vi "Fundamental Phasors.vi"(8 "error in (no error)":errorcluster, 10 "current waveform":waveform(dbl), 11 "voltage waveform":waveform(dbl)) -> (0 "error out":errorcluster, 1 "frequency":dbl, 2 "current fundamental vector":cdb, 3 "voltage fundamental vector":cdb)   [LabVIEW 2021]
uses:
  <vilib>/measure/matone.llb/Extract Single Tone Information 1 Chan.vi
  <vilib>/measure/NI_MAPro.lvlib
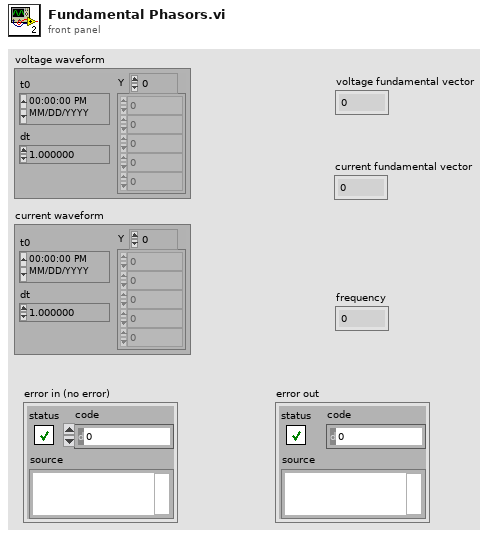
[diagram p1: front panel]
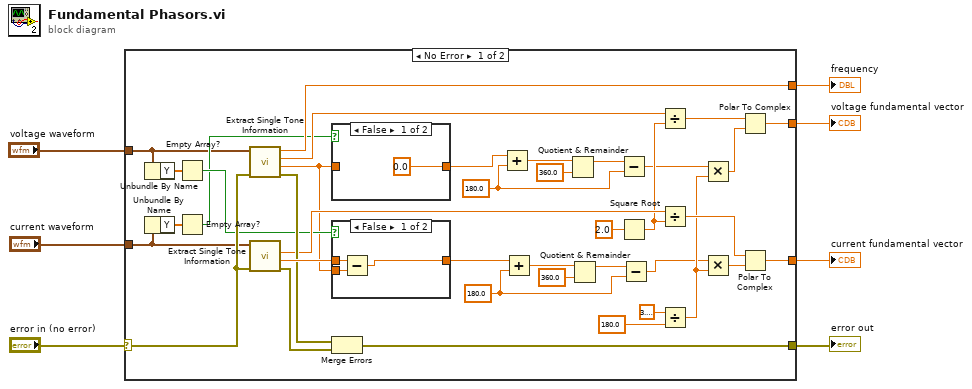
[diagram p0: block diagram]
diagram:
  n1 = case shown="No Error" "error in (no error)" {
    selector: "error in (no error)" -> [w40 w52]
    tunnel: "voltage waveform" -> [w20 _]
    tunnel: [w31 w52] -> w2
    tunnel: [w42 _] -> w6
    tunnel: [w41 _] -> w3
    tunnel: "current waveform" -> [w21 _]
    tunnel: [w34 _] -> w4
    frame No Error {
      w10 = 180.0 ("x")
      w16 = 180.0 ("x")
      n2 = Unbundle By Name(w20) -> ("Y"=w29:dbl[])
      n3 = Unbundle By Name(w21) -> ("Y"=w27:dbl[])
      n4 = Empty Array?(array=w29) -> (empty?=w28:bool)
      n5 = Empty Array?(array=w27) -> (empty?=w26:bool)
      n6 = call-poly <vilib>:"Extract Single Tone Information.vi"("error in (no error)"=w40, "time signal in"=w20) -> ("error out"=w32:errorcluster, "detected phase (deg)"=w25:dbl, "detected amplitude"=w43:dbl, "detected frequency"=w41:dbl)  [unwired: 2 in, 4 out]
      n7 = call-poly <vilib>:"Extract Single Tone Information.vi"("error in (no error)"=w40, "time signal in"=w21) -> ("error out"=w33:errorcluster, "detected phase (deg)"=w35:dbl, "detected amplitude"=w30:dbl)  [unwired: 2 in, 5 out]
      n8 = case shown="False" w26 {
        tunnel: [0.0 ("detected phase (deg)") w47] -> w14
        tunnel: w25 -> [_ w47]
        frame False {
          # "voltage phase = ref"
        }
        frame True {
          # "No current signal"
        }
      }
      n9 = case shown="False" w28 {
        tunnel: w35 -> [w50 w51]
        tunnel: [w49 w51] -> w9
        tunnel: w25 -> [w48 _]
        frame False {
          # "relative phase"
          n10 = Subtract(x=w50, y=w48) -> (x-y=w49:dbl)
        }
        frame True {
          # "No voltage signal"
        }
      }
      n11 = Merge Errors(w32, w33) -> (w31:errorcluster)
      n12 = Add(x=w14, y=w16) -> (x+y=w19:dbl)
      n13 = Add(x=w9, y=w10) -> (x+y=w13:dbl)
      n14 = Quotient & Remainder(x=w19, y=360.0) -> (x-y*floor(x/y)=w17:dbl)  [unwired: 1 out]
      n15 = Quotient & Remainder(x=w13, y=360.0) -> (x-y*floor(x/y)=w11:dbl)  [unwired: 1 out]
      n16 = Subtract(x=w17, y=w16) -> (x-y=w15:dbl)
      n17 = Square Root(x=2.0) -> (sqrt(x)=w24:dbl)
      n18 = Subtract(x=w11, y=w10) -> (x-y=w8:dbl)
      n19 = Divide(x=w43, y=w24) -> (x/y=w44:dbl)
      n20 = Divide(x=w30, y=w24) -> (x/y=w39:dbl)
      n21 = Divide(x=3.141592653589793, y=180.0) -> (x/y=w22:dbl)
      n22 = Multiply(x=w15, y=w22) -> (x*y=w45:dbl)
      n23 = Multiply(x=w8, y=w22) -> (x*y=w37:dbl)
      n24 = Polar To Complex(1:w45, 2:w44) -> (0:w42:cdb)
      n25 = Polar To Complex(1:w37, 2:w39) -> (0:w34:cdb)
    }
    frame Error {
    }
  }
  "voltage fundamental vector" <- w6
  "current fundamental vector" <- w4
  "error out" <- w2
  "frequency" <- w3
